vi "2D Look-Up Table (DBL Array).vi"(2 "LUT":dbl[][](array[numeric]) format="%.2f", 3 "Y Indexes (column)":dbl[](array[numeric]) format="%.2f", 4 "X Indexes (row)":dbl[](array[numeric]) format="%.2f") -> (1 "output points":dbl[](array[numeric]) format="%.2f")   [LabVIEW 2020, in "NI_AdvCtrl_nonlinear.lvlib"]
doc: "LabVIEW no longer supports this VI. You can obtain similar functionality by installing the LabVIEW Simulation Module.\n\nSearches for an element in a given 2D table that has a fractional x-index and y-index (interpolation)."
uses:
  <vilib>/addons/control/advanced/NI_AdvCtrl_nonlinear.lvlib
  <vilib>/addons/control/advanced/NI_AdvCtrl_continuous linear.lvlib
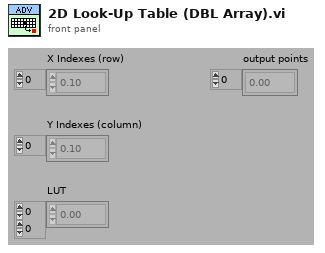
[diagram p1: front panel]
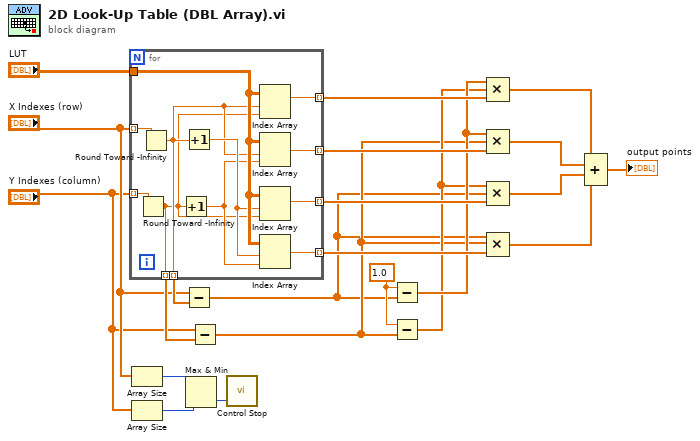
[diagram p0: block diagram]
diagram:
  w18 = 1.0 ("x")
  n1 = for {
    tunnel: "LUT" -> [w33]
    tunnel: "Y Indexes (column)" -> [w32] mode=indexing
    tunnel: "X Indexes (row)" -> [w31] mode=indexing
    tunnel: [w28] -> w20 mode=indexing
    tunnel: [w27] -> w19 mode=indexing
    tunnel: [w26] -> w17 mode=indexing
    tunnel: [w25] -> w16 mode=indexing
    tunnel: [w24] -> w15 mode=indexing
    tunnel: [w23] -> w14 mode=indexing
    n2 = Round Toward -Infinity(1:w32) -> (0:w27:dbl)
    n3 = Round Toward -Infinity(1:w31) -> (0:w28:dbl)
    n4 = Increment(x=w27) -> (x+1=w29:dbl)
    n5 = Increment(x=w28) -> (x+1=w30:dbl)
    n6 = Index Array(array=w33, index (row)=w28, index (col)=w27) -> (element=w26:dbl)
    n7 = Index Array(array=w33, index (row)=w28, index (col)=w29) -> (element=w24:dbl)
    n8 = Index Array(array=w33, index (row)=w30, index (col)=w27) -> (element=w25:dbl)
    n9 = Index Array(array=w33, index (row)=w30, index (col)=w29) -> (element=w23:dbl)
  }
  n10 = Array Size(array="X Indexes (row)") -> (size(s)=w6:i32)
  n11 = Array Size(array="Y Indexes (column)") -> (size(s)=w7:i32)
  n12 = Subtract(x="X Indexes (row)", y=w20) -> (x-y=w2:dbl[])
  n13 = Max & Min(x=w6, y=w7) -> (min(x,y)=w1:i32)  [unwired: 1 out]
  n14 = Subtract(x="Y Indexes (column)", y=w19) -> (x-y=w3:dbl[])
  n15 = call <vilib>:"Control Stop.vi"("error"=w1) -> ()  [unwired: 2 out]
  n16 = Subtract(x=w18, y=w2) -> (x-y=w5:dbl[])
  n17 = Subtract(x=w18, y=w3) -> (x-y=w4:dbl[])
  n18 = Compound Arithmetic op=MULTIPLY(w5, w4, w17) -> (w13:dbl[])
  n19 = Compound Arithmetic op=MULTIPLY(w5, w3, w15) -> (w11:dbl[])
  n20 = Compound Arithmetic op=MULTIPLY(w4, w2, w16) -> (w10:dbl[])
  n21 = Compound Arithmetic op=MULTIPLY(w2, w3, w14) -> (w12:dbl[])
  n22 = Compound Arithmetic op=ADD(w13, w11, w10, w12) -> (→"output points":dbl[])
